vi "Create.vi"() -> (0 "error out":errorcluster, 3 "BCReg":refnum<data-value>)   [LabVIEW 2014, in "BusController.lvlib" / "BCReg.lvclass"]
uses:
  BCReg.lvclass
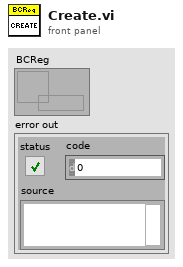
[diagram p1: front panel]
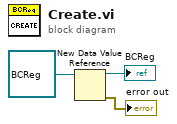
[diagram p0: block diagram]
diagram:
  n1 = New Data Value Reference(data value=refnum<class "BCReg.lvclass"> refnum ("BusController.lvlib:BCReg.lvclass")) -> (data value reference=→"BCReg":refnum<data-value>, error out=→"error out":errorcluster)  [unwired: 1 in]
